vi "TimeInfoOPEN.vi"(7 "error in (no error)":errorcluster, 9 "Minor Time":u32, 10 "Major Time":u32) -> (0 "Date":cluster{"Date":string, "Error":string}, 1 "Open":cluster{"Time":string, "Error":string})   [LabVIEW 2015]
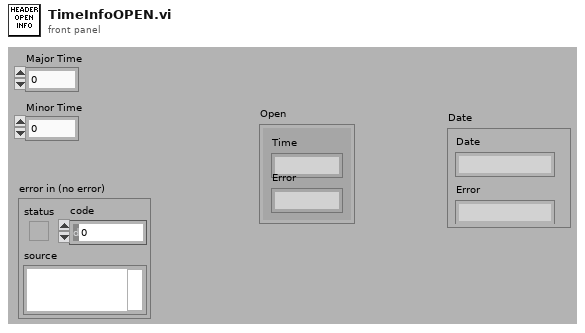
[diagram p1: front panel]
types:
  T1 = cluster{"  Open Time":string, "Open Error":string}
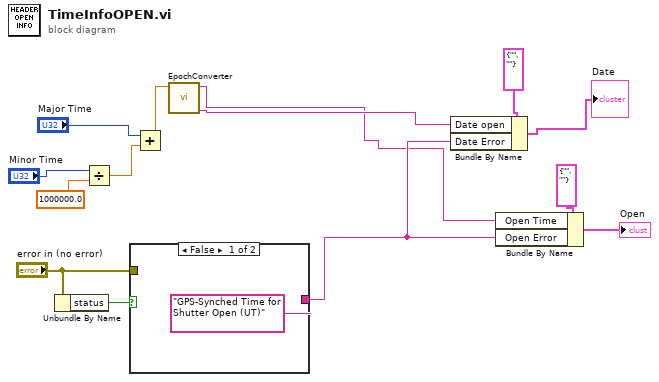
[diagram p0: block diagram]
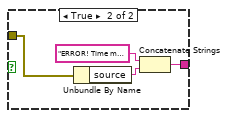
[diagram p2: hidden frame]
diagram:
  n1 = Unbundle By Name("error in (no error)") -> ("status"=w14:bool)
  n2 = Divide(x="Minor Time", y=1000000.0) -> (x/y=w3:dbl)
  n3 = case shown="False" w14 {
    tunnel: "error in (no error)" -> [_ w19]
    tunnel: ["GPS-Synched Time for Shutter Open (UT)" w18] -> w8
    frame False {
    }
    frame True {
      n4 = Unbundle By Name(w19) -> ("source"=w17:string)
      n5 = Concatenate Strings("ERROR! Time may be Invalid.  Source: ", w17) -> (w18:string)
    }
  }
  n6 = Add(x="Major Time", y=w3) -> (x+y=w2:dbl)
  n7 = call "EpochConverter.vi"("Epoch time"=w2) -> ("Date"=w10:string, "String"=w1:string)  [unwired: 9 in]
  n8 = Bundle By Name(cluster=cluster{"Date open":string, "Date Error":string} {"Date open"="", "Date Error"=""}, "Date open"=w10, "Date Error"=w8) -> (→"Date":cluster{"Date open":string, "Date Error":string})
  n9 = Bundle By Name(cluster=T1 {"  Open Time"="", "Open Error"=""}, "Open Time"=w1, "Open Error"=w8) -> (→"Open":T1)
